vi "global.vi"() -> ()   [LabVIEW 2019]
panel:
  in  "Repeat Trial":bool
  out "Total Trials":i32
  out "Trial":i32
  out "Green Light":bool
  out "Red Light":bool
  in  "Choice Equal":bool
  in  "Choice 2":bool
  in  "Choice 1":bool
  out "Sound number":string
  in  "Start":bool
  in  "stop":bool
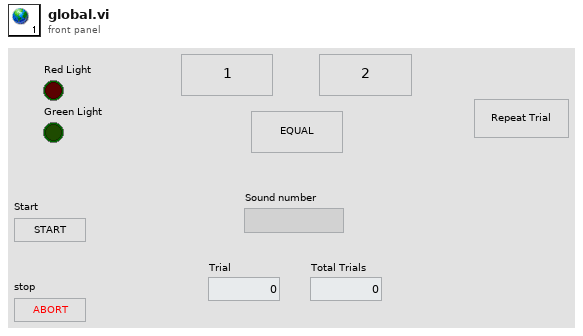
[diagram p1: front panel]
diagram:
